vi "Master network read write.vi"(7 "Modbus master in":refnum<class "Modbus Master.lvclass">, 8 "error in (no error)":errorcluster, 9 "transmission data unit in":refnum<class "Transmission Data Unit.lvclass">, 10 "network master in":refnum<class "Network Master.lvclass">, 11 "Modbus data unit in":refnum<class "Modbus Data Unit.lvclass">) -> (0 "error out":errorcluster, 2 "PDU valid?":bool, 3 "Modbus data unit out":refnum<class "Modbus Data Unit.lvclass">, 5 "Modbus master out":refnum<class "Modbus Master.lvclass">)   [LabVIEW 2021, in "Modbus Master.lvclass"]
doc: "This VI allows a mutex for the master API without restricting any other functions. This mutex is currently unimplemented."
uses:
  Modbus Master.lvclass
  Network Protocol/Network Master/Network Master.lvclass
  D:/my_projects/projects/Algorithms/Labview/21/Modbus_v1/Network Protocol/Network Protocol.lvclass
  Transmission Data Unit/Transmission Data Unit.lvclass
  Modbus Data Unit/Modbus Data Unit.lvclass
  Modbus Master.lvclass/Modbus Master.ctl
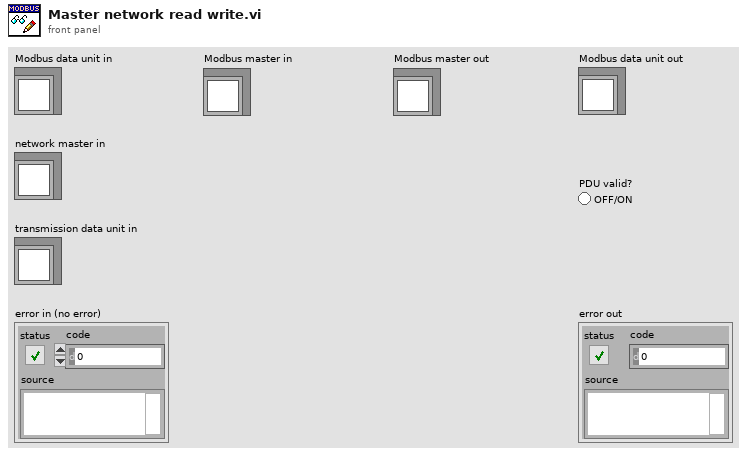
[diagram p1: front panel]
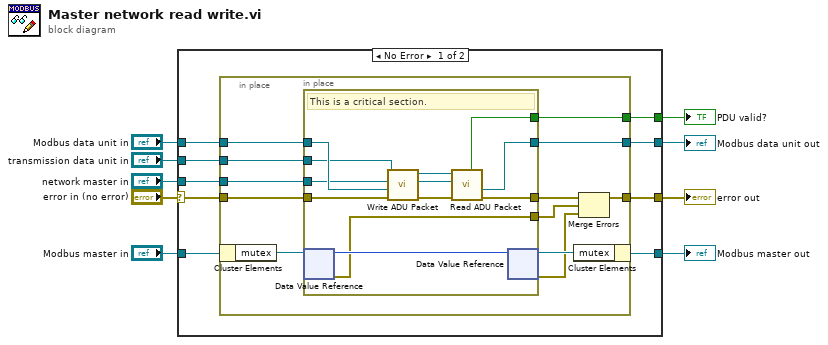
[diagram p0: block diagram]
diagram:
  n1 = case shown="No Error" "error in (no error)" {
    selector: "error in (no error)" -> [w10 w43]
    tunnel: "Modbus master in" -> [w18 w44]
    tunnel: [w17 w44] -> w8
    tunnel: "Modbus data unit in" -> [w16 w45]
    tunnel: "transmission data unit in" -> [w15 _]
    tunnel: "network master in" -> [w14 _]
    tunnel: [w13 w45] -> w4
    tunnel: [w12 w43] -> w3
    tunnel: [w11 _] -> w2
    frame No Error {
      n2 = in-place {
        in-place-border: w10 -> [w29]
        in-place-border: w16 -> [w28]
        in-place-border: w15 -> [w26]
        in-place-border: w14 -> [w25]
        in-place-border: [w24] -> w13
        in-place-border: [w23] -> w12
        in-place-border: [w22] -> w11
        n3 = in-place-cluster #1(w18) -> ("mutex"=w30:refnum<data-value>)
        n4 = in-place {
          in-place-border: w29 -> [w38]
          in-place-border: w28 -> [w37]
          in-place-border: w26 -> [w36]
          in-place-border: w25 -> [w34]
          in-place-border: [w35] -> w21
          in-place-border: [w33] -> w24
          in-place-border: [w32] -> w22
          in-place-border: [w31] -> w20
          # "This is a critical section."
          n5 = in-place-dvr #2(w30) -> (w39:u8, w31:errorcluster)
          n6 = call-dynamic "Write ADU Packet.vi"("error in"=w38, "modbus data unit"=w37, "protocol layer"=w34, "transmission data unit in"=w36) -> ("error out"=w41:errorcluster, "protocol layer out"=w42:refnum<class "Network Protocol.lvclass">, "transmission data unit out"=w40:refnum<class "Transmission Data Unit.lvclass">)  [unwired: 5 in]
          n7 = call-dynamic "Read ADU Packet.vi"("error in"=w41, "protocol layer"=w42, "transmission data unit in"=w40) -> ("error out"=w35:errorcluster, "modbus data unit"=w33:refnum<class "Modbus Data Unit.lvclass">, "PDU Valid?"=w32:bool)  [unwired: 4 in, 2 out]
          n8 = in-place-dvr #2(w39) -> (w27:refnum<data-value>, w19:errorcluster)
        }
        n9 = in-place-cluster #1("mutex"=w27) -> (w17:refnum<class "Modbus Master.lvclass">)
        n10 = Merge Errors(w21, w20, w19) -> (w23:errorcluster)
      }
    }
    frame Error {
    }
  }
  "Modbus data unit out" <- w4
  "Modbus master out" <- w8
  "error out" <- w3
  "PDU valid?" <- w2
